vi "Rx Async.vi"(8 "error in (no error)":errorcluster, 10 "Dispatcher Interface in":refnum<class "Dispatcher Interface.lvclass">, 11 "Plugin in":refnum<class "Plugin.lvclass">) -> (0 "error out":errorcluster, 2 "Dispatcher Interface out":refnum<class "Dispatcher Interface.lvclass">, 3 "Plugin out":refnum<class "Plugin.lvclass">)   [LabVIEW 2017, in "DSF Core.lvlib" / "Plugin.lvclass"]
uses:
  Plugin.lvclass
  Interface/Dispatcher/Dispatcher Interface.lvclass
  Plugin.lvclass/Plugin.ctl
  Interface/Dispatcher/Command.ctl
  Transfer Group/Transfer Group.lvclass
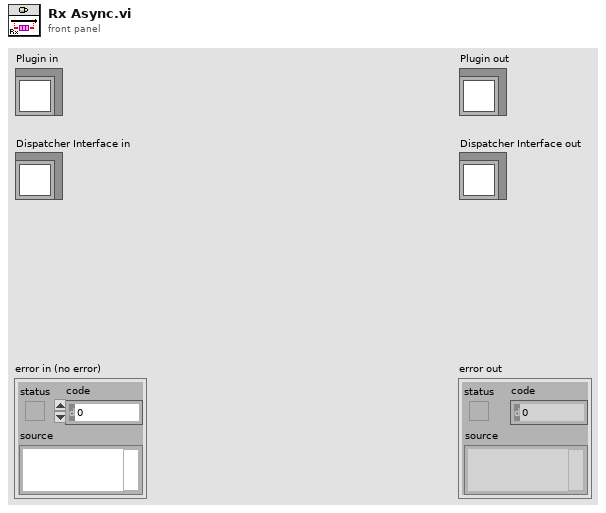
[diagram p1: front panel]
types:
  T1 = typedef "DSF Core.lvlib/Dispatcher Interface.lvclass/Command.ctl" = enum8{"Idle", "Start", "Rx", "Tx", "Set Inline Buffer", "Shutdown", "Error"}
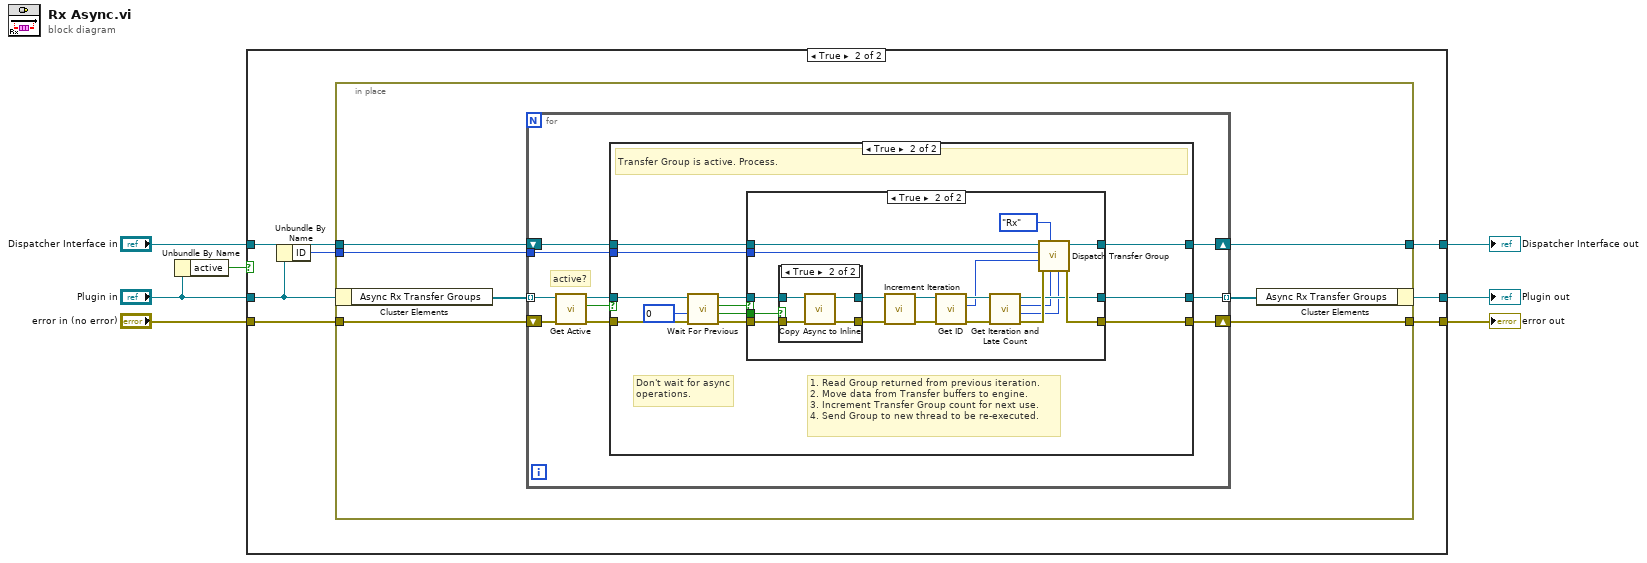
[diagram p0: block diagram]
diagram:
  n1 = Unbundle By Name("Plugin in") -> ("active"=w1:bool)
  n2 = case shown="True" w1 {
    tunnel: "error in (no error)" -> [w8 w17]
    tunnel: [w8 w16] -> w6
    tunnel: [w10 w15] -> w5
    tunnel: "Dispatcher Interface in" -> [w9 w14]
    tunnel: [w9 w13] -> w3
    tunnel: "Plugin in" -> [w10 w12]
    frame False {
    }
    frame True {
      n3 = Unbundle By Name(w12) -> ("ID"=w11:i32)
      n4 = in-place {
        in-place-border: w17 -> [w24]
        in-place-border: [w23] -> w16
        in-place-border: w14 -> [w20]
        in-place-border: [w19] -> w13
        in-place-border: w11 -> [w18]
        n5 = in-place-cluster #1(w12) -> ("Async Rx Transfer Groups"=w22:refnum<class "Transfer Group.lvclass">[])
        n6 = for {
          tunnel: w22 -> [w27] mode=indexing
          shift-right: [w33] -> w23
          shift-left: w24 -> [w32]
          tunnel: [w31] -> w21 mode=indexing
          shift-right: [w29] -> w19
          shift-left: w20 -> [w30]
          tunnel: w18 -> [w28]
          # "active?"
          n7 = call "Get Active.vi"("Transfer Group in"=w27) -> ("active"=w25:bool, "Transfer Group out"=w26:refnum<class "Transfer Group.lvclass">)  [unwired: 9 in]
          n8 = case shown="True" w25 {
            tunnel: [w36 w38] -> w33
            tunnel: w32 -> [w36 w47]
            tunnel: w26 -> [w35 w48]
            tunnel: [w35 w39] -> w31
            tunnel: w30 -> [w34 w42]
            tunnel: [w34 w43] -> w29
            tunnel: w28 -> [_ w41]
            frame False {
              # "Transfer Group is not active. Skip."
            }
            frame True {
              # "Don't wait for async operations."
              # "1. Read Group returned from previous iteration.\n2. Move data from Transfer buffers to engine.\n3. Increment Transfer Group count for next use.\n4. Send Group to new thread to be re-executed."
              # "Transfer Group is active. Process."
              n9 = call "Wait For Previous.vi"("error in (no error)"=w47, "timeout in ms (0)"=0, "Transfer Group in"=w48) -> ("error out"=w44:errorcluster, "move data"=w37:bool, "ready for next"=w40:bool, "Transfer Group out"=w45:refnum<class "Transfer Group.lvclass">)  [unwired: 5 in]
              n10 = case shown="True" w40 {
                tunnel: w45 -> [w51 w69]
                tunnel: [w51 w58] -> w39
                tunnel: [w50 w59] -> w38
                tunnel: w44 -> [w50 w68]
                tunnel: [w49 w56] -> w43
                tunnel: w42 -> [w49 w55]
                tunnel: w41 -> [_ w54]
                tunnel: w37 -> [_ w53]
                frame False {
                }
                frame True {
                  n11 = case shown="True" w53 {
                    tunnel: w69 -> [w71 w75]
                    tunnel: w68 -> [w70 w74]
                    tunnel: [w71 w73] -> w61
                    tunnel: [w70 w72] -> w60
                    frame False {
                    }
                    frame True {
                      n12 = call "Copy Async to Inline.vi"("error in (no error)"=w74, "Transfer Group in"=w75) -> ("error out"=w72:errorcluster, "Transfer Group out"=w73:refnum<class "Transfer Group.lvclass">)  [unwired: 8 in]
                    }
                  }
                  n13 = call "Increment Iteration.vi"("error in (no error)"=w60, "Transfer Group in"=w61) -> ("error out"=w65:errorcluster, "Transfer Group out"=w67:refnum<class "Transfer Group.lvclass">)  [unwired: 8 in]
                  n14 = call "Get ID.vi"("Transfer Group in"=w67) -> ("id"=w64:i32, "Transfer Group out"=w66:refnum<class "Transfer Group.lvclass">)  [unwired: 9 in]
                  n15 = call "Get Iteration and Late Count.vi"("error in (no error)"=w65, "Transfer Group in"=w66) -> ("error out"=w63:errorcluster, "late count"=w52:i32, "iteration"=w57:u64, "Transfer Group out"=w58:refnum<class "Transfer Group.lvclass">)  [unwired: 6 in]
                  n16 = call "Dispatch Transfer Group.vi"("Late Count"=w52, "Iteration"=w57, "command"=Command."Rx", "error in (no error)"=w63, "Transfer Group ID"=w64, "Plugin ID"=w54, "Dispatcher Interface in"=w55) -> ("error out"=w59:errorcluster, "Dispatcher Interface out"=w56:refnum<class "Dispatcher Interface.lvclass">)  [unwired: 3 in]
                }
              }
            }
          }
        }
        n17 = in-place-cluster #1("Async Rx Transfer Groups"=w21) -> (w15:refnum<class "Plugin.lvclass">)
      }
    }
  }
  "error out" <- w6
  "Plugin out" <- w5
  "Dispatcher Interface out" <- w3
